vi "FindLocation.vi"(0 "Motion Settings":T1={"No Motion?"=FALSE, "Motion System"=enum."NI 735x", "Motion Bd ID"=1, "Motion Profile"="SMAC1", "# Axis"=1, "Reverse Z axis?"=TRUE, "SMAC Axis"=0, "scan pair"=enum."y-(x) scan", "RT fps"=6.0, "Steps per mm"=[1000, 1000, 1000, 1000], "Motor Parameters"={"velocity ct/s"=[10000.0, 10000.0, 10000.0, 50000.0], "accel ct/s^2"=[50000.0, 50000.0, 50000.0, 200000.0]}, "One Way Scan"=FALSE, "Reverse One Way Scan"=FALSE, "Global Position (mm)"=[], "Plane"=0, "Distance between\nscan lines (um)"=0.0, "Distance between\nscan planes (um)"=0.0, "number of scan planes"=1, "Total steps in line"=0, "Xtra plane\ndistance  (um)"=100, "Xtra planes "=1, "Add Axis"=FALSE, "overshoot cts"=200, "BKPT Shift"=0, "Scan Start Time (ms)"=0, "ESP VISA"="GPIB::1::INSTR", "3rd Axis"=1, "GL Ref Out"=refnum, "Galil Address"=""} {"3rd Axis" items=["x", "y", "z", "w"]; "Xtra planes" min=1; "Xtra plane\ndistance  (um)" min=0; "Distance between\nscan planes (um)" format="%.2f"; "Distance between\nscan lines (um)" format="%.2f"; "SMAC Axis" items=["None"=0, "Axis 1"=1, "Axis 2"=2, "Axis 3"=3, "Axis 4"=4, "Axis 5"=5, "Axis 6"=6, "Axis 7"=7, "Axis 8"=8, "Vector Space 1"=17, "Vector Space 2"=18, "Vector Space 3"=19, "Vector Space 4"=20]; "Motion Bd ID" min=1 max=32 step=1}, 1 "Wait for Motion Complete":bool=TRUE, 2 "error in (no error)":errorcluster) -> (3 "Motion Settings Out":T1={"No Motion?"=FALSE, "Motion System"=enum."NI 735x", "Motion Bd ID"=1, "Motion Profile"="SMAC1", "# Axis"=1, "Reverse Z axis?"=TRUE, "SMAC Axis"=0, "scan pair"=enum."y-(x) scan", "RT fps"=6.0, "Steps per mm"=[1000, 1000, 1000, 1000], "Motor Parameters"={"velocity ct/s"=[10000.0, 10000.0, 10000.0, 50000.0], "accel ct/s^2"=[50000.0, 50000.0, 50000.0, 200000.0]}, "One Way Scan"=FALSE, "Reverse One Way Scan"=FALSE, "Global Position (mm)"=[], "Plane"=0, "Distance between\nscan lines (um)"=0.0, "Distance between\nscan planes (um)"=0.0, "number of scan planes"=1, "Total steps in line"=0, "Xtra plane\ndistance  (um)"=100, "Xtra planes "=1, "Add Axis"=FALSE, "overshoot cts"=200, "BKPT Shift"=0, "Scan Start Time (ms)"=0, "ESP VISA"="GPIB::1::INSTR", "3rd Axis"=1, "GL Ref Out"=refnum, "Galil Address"=""} {"3rd Axis" items=["x", "y", "z", "w"]; "Xtra planes" min=1; "Xtra plane\ndistance  (um)" min=0; "Distance between\nscan planes (um)" format="%.2f"; "Distance between\nscan lines (um)" format="%.2f"; "SMAC Axis" items=["None"=0, "Axis 1"=1, "Axis 2"=2, "Axis 3"=3, "Axis 4"=4, "Axis 5"=5, "Axis 6"=6, "Axis 7"=7, "Axis 8"=8, "Vector Space 1"=17, "Vector Space 2"=18, "Vector Space 3"=19, "Vector Space 4"=20]; "Motion Bd ID" min=1 max=32 step=1}, 4 "location (mm)":dbl[](array[numeric]), 5 "Bd ID Out":u8, 6 "error out":errorcluster)   [LabVIEW 2022 SP3]
uses:
  MotionParameters.ctl
  MotionSys.ctl
  -MotionRoutines/ScanAxis.ctl
  -MotionRoutines/3rdAxis.ctl
panel:
  # "1-D and 2-D B scan settings"
  # "1-D and 2-D B scan settings"
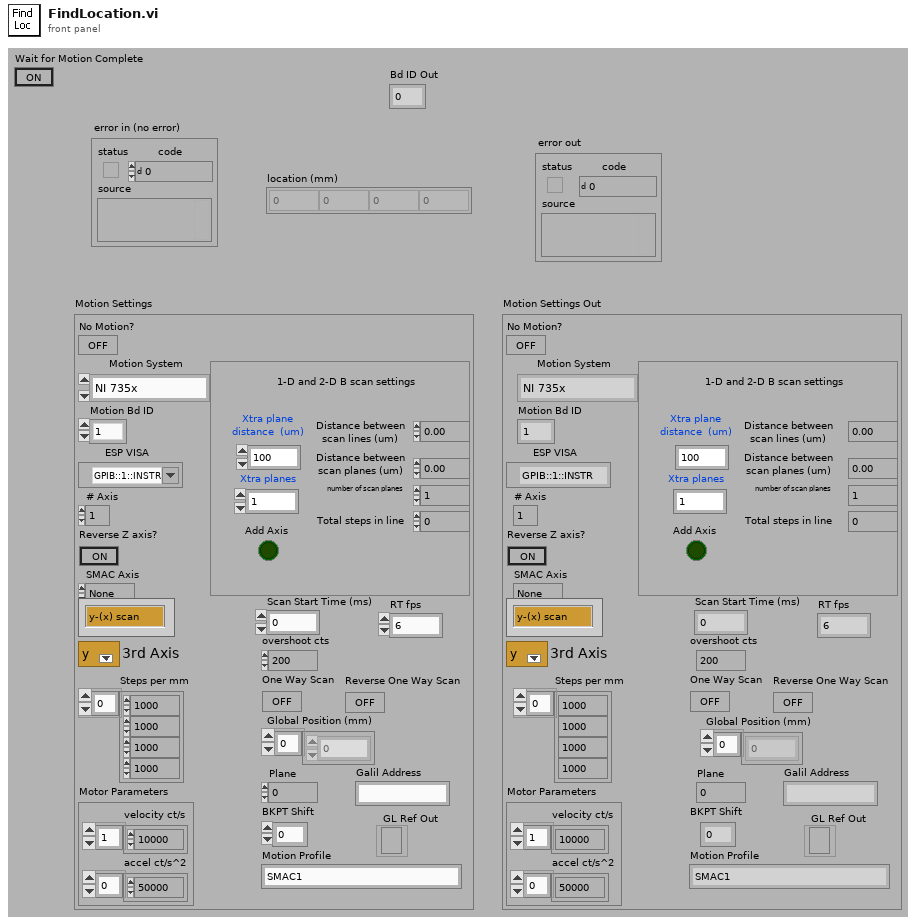
[diagram p1: front panel]
types:
  T1 = typedef "MotionParameters.ctl" = cluster{"No Motion?":bool, "Motion System":T2, "Motion Bd ID":u8, "Motion Profile":string, "# Axis":i8, "Reverse Z axis?":bool, "SMAC Axis":u16, "scan pair":T3, "RT fps":sgl, "Steps per mm":i32[], "Motor Parameters":cluster{"velocity ct/s":dbl[], "accel ct/s^2":dbl[]}, "One Way Scan":bool, "Reverse One Way Scan":bool, "Global Position (mm)":dbl[], "Plane":i32, "Distance between\nscan lines (um)":sgl, "Distance between\nscan planes (um)":sgl, "number of scan planes":i32, "Total steps in line":i32, "Xtra plane\ndistance  (um)":i32, "Xtra planes ":i32, "Add Axis":bool, "overshoot cts":i32, "BKPT Shift":i32, "Scan Start Time (ms)":u32, "ESP VISA":refnum<visa-resource-name>, "3rd Axis":T4, "GL Ref Out":refnum<k7>, "Galil Address":string}
  T2 = typedef "MotionSys.ctl" = enum16{"MM3000", "NI 735x", "Newport ESP", "No Motion Card", "Galil"}
  T3 = typedef "ScanAxis.ctl" = enum16{"y-(x) scan", "x-(y) scan", "z-(x) scan", "z-(y) scan", "y-(z) scan", "x-(z) scan", "w-(x) scan", "w-(y) scan", "w-(z) scan", "x-(w) scan", "y-(w) scan", "z-(w) scan"}
  T4 = typedef "3rdAxis.ctl" = u16
  T5 = cluster{"Reserved":bool, "Axis #1 Move Complete":bool, "Axis #2 Move Complete":bool, "Axis #3 Move Complete":bool, "Axis #4 Move Complete":bool, "Axis #5 Move Complete":bool, "Axis #6 Move Complete":bool, "Axis #7 Move Complete":bool, "Axis #8 Move Complete":bool, "Axis #9 MoveComplete":bool, "Axis #10 Move Complete":bool, "Axis #11 Move Complete":bool, "Axis #12 Move Complete":bool, "Status #13":bool, "Status #14":bool, "Status #15":bool}
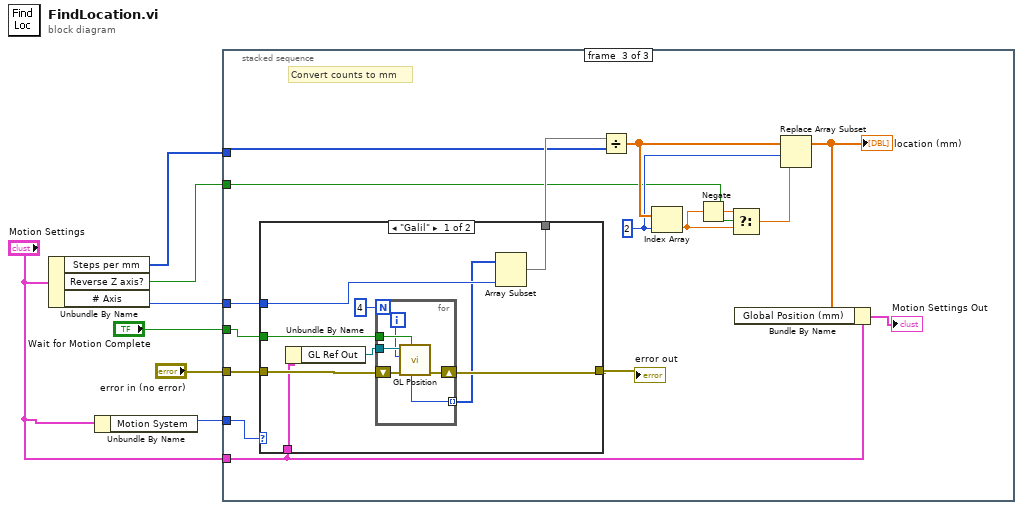
[diagram p0: block diagram]
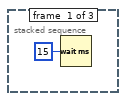
[diagram p2: hidden frame]
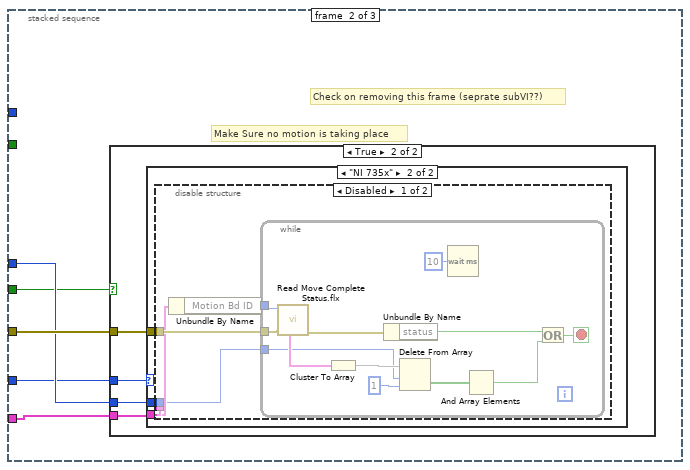
[diagram p3: hidden frame]
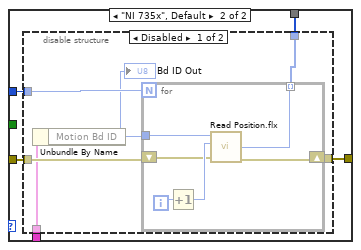
[diagram p7: hidden frame]
diagram:
  n1 = Unbundle By Name("Motion Settings") -> ("Steps per mm"=w5:i32[], "Reverse Z axis?"=w4:bool, "# Axis"=w6:i8)
  n2 = Unbundle By Name("Motion Settings") -> ("Motion System"=w1:T2)
  n3 = stacked-sequence {
    tunnel: "error in (no error)" -> [_ w13 w48]
    tunnel: w6 -> [_ w12 w47]
    tunnel: w5 -> [_ _ w43]
    tunnel: w4 -> [_ _ w42]
    tunnel: "Motion Settings" -> [_ w9 w37]
    tunnel: "Wait for Motion Complete" -> [_ w11 w38]
    tunnel: w1 -> [_ w10 w39]
    frame #0 {
      n4 = Wait (ms)(milliseconds to wait=15) -> ()  [unwired: 1 out]
    }
    frame #1 {
      # "Check on removing this frame (seprate subVI??)"
      # "Make Sure no motion is taking place"
      n5 = case shown="True" w11 {
        tunnel: w13 -> [_ w17]
        tunnel: w12 -> [_ w16]
        tunnel: w10 -> [_ w15]
        tunnel: w9 -> [_ w14]
        frame False {
        }
        frame True {
          n6 = case shown="\"NI 735x\"" w15 {
            tunnel: w17 -> [_ w20]
            tunnel: w16 -> [_ w18]
            tunnel: w14 -> [_ w19]
            frame "Galil", Default {
            }
            frame "NI 735x" {
              n7 = disable-structure shown="Disabled" {
                disable-tunnel: w20 -> [w24 _]
                disable-tunnel: w19 -> [w23 _]
                disable-tunnel: w18 -> [w21 _]
                frame Disabled {
                  n8 = Unbundle By Name(w23) -> ("Motion Bd ID"=w22:u8)
                  n9 = while {
                    tunnel: w24 -> [w33]
                    tunnel: w21 -> [w27]
                    tunnel: w22 -> [w25]
                    stop <- w35 stop-if-true
                    n10 = call <vilib>:"Read Move Complete Status.flx"("error in (no error)"=w33, "Board ID"=w25) -> ("error out"=w32:errorcluster, "Move Complete Status"=w31:T5)  [unwired: 1 in, 4 out]
                    n11 = Cluster To Array(cluster=w31) -> (array=w29:bool[])
                    n12 = Unbundle By Name(w32) -> ("status"=w36:bool)
                    n13 = Delete From Array(array=w29, length=w27, index=1) -> (deleted portion=w26:bool[])  [unwired: 1 out]
                    n14 = Wait (ms)(milliseconds to wait=10) -> ()  [unwired: 1 out]
                    n15 = And Array Elements(Boolean array=w26) -> (logical AND=w30:bool)
                    n16 = Or(x=w36, y=w30) -> (x .or. y?=w35:bool)
                  }
                }
                frame Enabled {
                }
              }
            }
          }
        }
      }
    }
    frame #2 {
      w45 = 2 ("Axis")
      # "Convert counts to mm"
      n17 = case shown="\"Galil\"" w39 {
        tunnel: [w61 w72] -> w52
        tunnel: [w58 w71] -> w49
        tunnel: w48 -> [w60 w70]
        tunnel: w47 -> [w59 w69]
        tunnel: w38 -> [w57 _]
        tunnel: w37 -> [w56 w68]
        frame "Galil" {
          n18 = Unbundle By Name(w56) -> ("GL Ref Out"=w55:refnum<k7>)
          n19 = for {
            N: 4 -> [_]
            tunnel: w57 -> [w65]
            tunnel: w55 -> [w64]
            shift-right: [w67] -> w61
            shift-left: w60 -> [w66]
            tunnel: [w63] -> w54 mode=indexing
            i -> [w62]
            n20 = call "GL Position.vi"("Wait for Motion Complete"=w65, "error in (no error)"=w66, "Axis"=w62, "Galil.IGalil"=w64) -> ("error out"=w67:errorcluster, "Axis Position"=w63:i32)  [unwired: 2 in, 2 out]
          }
          n21 = Array Subset(array=w54, length=w59) -> (w58:i32[])  [unwired: 1 in]
        }
        frame "NI 735x", Default {
          n22 = disable-structure shown="Disabled" {
            disable-tunnel: [w78 _] -> w72
            disable-tunnel: [w77 _] -> w71
            disable-tunnel: w70 -> [w76 _]
            disable-tunnel: w69 -> [w75 _]
            disable-tunnel: w68 -> [w74 _]
            frame Disabled {
              n23 = Unbundle By Name(w74) -> ("Motion Bd ID"=w73:u8)
              "Bd ID Out" <- w73
              n24 = for {
                N: w75 -> [_]
                shift-right: [w80] -> w78
                shift-left: w76 -> [w82]
                tunnel: [w81] -> w77 mode=indexing
                tunnel: w73 -> [w79]
                i -> [w84]
                n25 = Increment(x=w84) -> (x+1=w83:i32)
                n26 = call <vilib>:"Read Position.flx"("error in (no error)"=w82, "Axis"=w83, "Board ID"=w79) -> ("error out"=w80:errorcluster, "Position"=w81:i32)  [unwired: 5 out]
              }
            }
            frame Enabled {
            }
          }
        }
      }
      "error out" <- w52
      n27 = Divide(x=w49, y=w43) -> (x/y=w46:dbl[])
      n28 = Index Array(array=w46, index=w45) -> (element=w50:dbl)
      n29 = Negate(x=w50) -> (-x=w51:dbl)
      n30 = Select(t=w51, s=w42, f=w50) -> (s? t:f=w44:dbl)
      n31 = Replace Array Subset(array=w46, new element=w44, index=w45) -> (w41:dbl[])
      "location (mm)" <- w41
      n32 = Bundle By Name(cluster=w37, "Global Position (mm)"=w41) -> (→"Motion Settings Out":T1)
    }
  }
